vi "Write Auto-Launch Nested Models.vi"(6 "Confirm Shutdown? (T)":bool=TRUE, 9 "Auto-stop? (T)":bool=TRUE, 10 "Auto-Launch Nested Models":refnum<class "IModel.lvclass">[](array[class]), 11 "IModel In":refnum<class "IModel.lvclass">) -> (3 "IModel Out":refnum<class "IModel.lvclass">)   [LabVIEW 2017, in "IModel.lvlib" / "IModel.lvclass"]
uses:
  <vilib>/gpm_packages/@cs/mva-core/Source/IModel/IModel/IModel.lvclass
  <vilib>/gpm_packages/@cs/mva-core/Source/IModel/IModel/IModel.lvclass/IModel.ctl
  <vilib>/gpm_packages/@cs/mva-core/Source/IModel/IModel Messages/Auto-Launch Models Msg/Auto-Launch Models Msg.lvclass
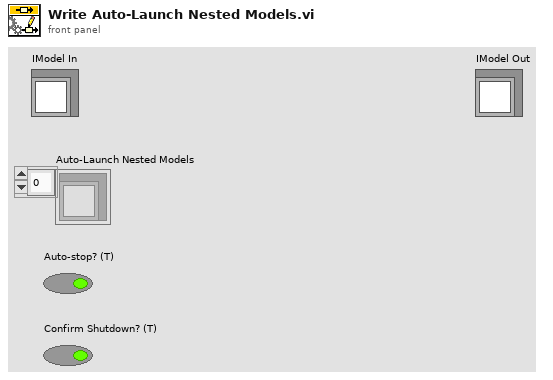
[diagram p1: front panel]
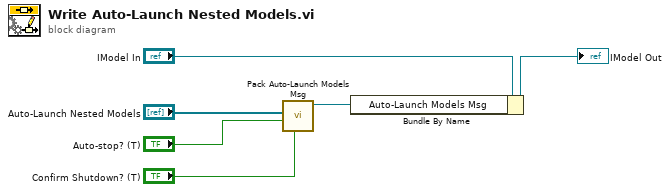
[diagram p0: block diagram]
diagram:
  n1 = call <vilib>:"Pack Auto-Launch Models Msg.vi"("Confirm Shutdown? (T)"="Confirm Shutdown? (T)", "Auto-stop? (T)"="Auto-stop? (T)", "Models"="Auto-Launch Nested Models") -> ("Launch Nested Models Msg"=w4:refnum<class "Auto-Launch Models Msg.lvclass">)  [unwired: 8 in]
  n2 = Bundle By Name(cluster="IModel In", "Auto-Launch Models Msg"=w4) -> (→"IModel Out":refnum<class "IModel.lvclass">)
